vi "get _g4_time.vi"(11 "Line in":string) -> (3 "Time to wait":u32)   [LabVIEW 2017, in "labview-standard-library.lvlib" / "automode-scripting.lvlib"]
uses:
  automode-scripting.lvlib
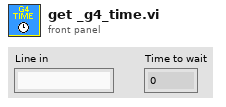
[diagram p1: front panel]
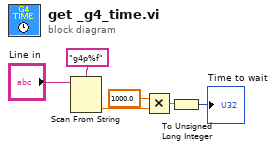
[diagram p0: block diagram]
diagram:
  n1 = Scan From String(format string="g4p%f", input string="Line in") -> (output 1=w2:dbl)  [unwired: 3 in, 3 out]
  n2 = Multiply(x=1000.0, y=w2) -> (x*y=w4:dbl)
  n3 = To Unsigned Long Integer(number=w4) -> (unsigned 32bit integer=→"Time to wait":u32)
